vi "board.failure.vi"(8 "error in (no error)":errorcluster, 11 "Game Board in":refnum<class "Game Board.lvclass">) -> (0 "error out":errorcluster, 2 "Fail":bool, 3 "Game Board out":refnum<class "Game Board.lvclass">)   [LabVIEW 2020, in "Game Board.lvclass"]
uses:
  Game Board.lvclass
  Game Board.lvclass/Game Board.ctl
  Snake/Snake.lvclass/Snake.ctl
  Snake/Snake.lvclass
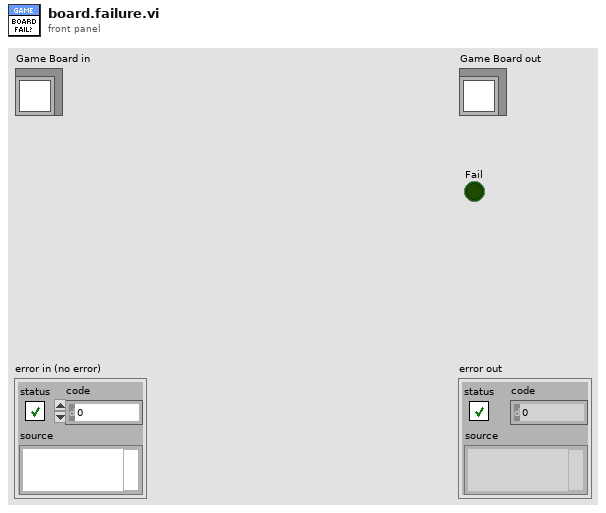
[diagram p1: front panel]
types:
  T1 = typedef "Coordinates.ctl" = cluster{"X":i32, "Y":i32}
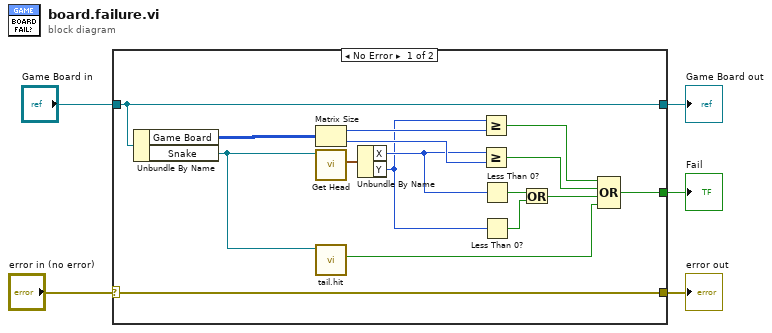
[diagram p0: block diagram]
diagram:
  n1 = case shown="No Error" "error in (no error)" {
    selector: "error in (no error)" -> [w21 w23]
    tunnel: [w21 w23] -> w4
    tunnel: [w20 w22] -> w2
    tunnel: "Game Board in" -> [w20 w22]
    tunnel: [w13 _] -> w1
    frame No Error {
      n2 = Unbundle By Name(w20) -> ("Game Board"=w17:u32[][], "Snake"=w7:refnum<class "Snake.lvclass">)
      n3 = Matrix Size(0:w17) -> (1:w11:i32, 2:w12:i32)
      n4 = call "Get Head.vi"("Snake in"=w7) -> ("Coordinates"=w10:T1)  [unwired: 10 in]
      n5 = call "tail.hit.vi"("Snake in"=w7) -> ("Tail Hit!?"=w6:bool)  [unwired: 8 in, 2 out]
      n6 = Unbundle By Name(w10) -> ("X"=w9:i32, "Y"=w8:i32)
      n7 = Greater Or Equal?(x=w8, y=w11) -> (x >= y?=w16:bool)
      n8 = Greater Or Equal?(x=w9, y=w12) -> (x >= y?=w15:bool)
      n9 = Less Than 0?(x=w9) -> (x < 0?=w19:bool)
      n10 = Less Than 0?(x=w8) -> (x < 0?=w18:bool)
      n11 = Or(x=w19, y=w18) -> (x .or. y?=w14:bool)
      n12 = Compound Arithmetic op=OR(w16, w15, w14, w6) -> (w13:bool)
    }
    frame Error {
    }
  }
  "error out" <- w4
  "Game Board out" <- w2
  "Fail" <- w1
